vi "Event-Camera.vi"(5 "Menu ref.":refnum<k9>, 7 "Camera":T1, 8 "error in (no error)":errorcluster, 10 "Data ref. in":refnum<data-value>, 11 "UI ref. in":refnum<data-value>) -> (0 "error out":errorcluster, 2 "Data ref.":refnum<data-value>, 3 "UI ref.":refnum<data-value>)   [LabVIEW 2013, in "CameraVision.lvlib" / "CV-UI.lvclass"]
uses:
  CV-UI.lvclass
  Main/CV-Main.lvclass
  Camera-selector.ctl
  CV-UI.lvclass/CV-UI.ctl
  Main/Main-actions.ctl
  Read Camera.vi
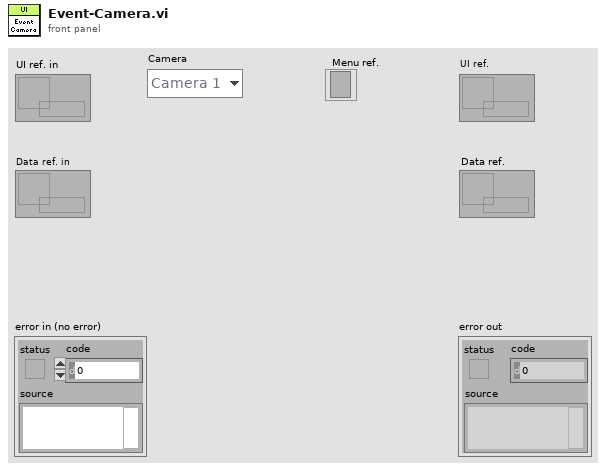
[diagram p1: front panel]
types:
  T1 = typedef "CameraVision.lvlib/CV-UI.lvclass/Camera-selector.ctl" = enum16{"Camera 1", "Camera 2"}
  T2 = typedef "CameraVision.lvlib/CV-Main.lvclass/Main-actions.ctl" = enum16{"Idle", "Initialize", "Load defaults", "Update settings", "Check settings", "Save settings", "Save settings with dialog", "Load settings", "Load data", "Activate", "Start", "Wait for start signal", "Acquire & process", "Iterate", "Stop", "Refresh display", "Refresh status", "View camera settings", "View grabber settings", "Exit"}
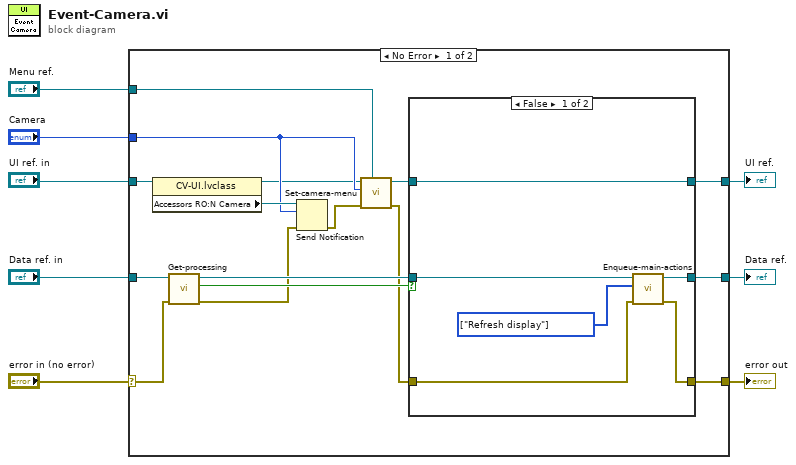
[diagram p0: block diagram]
diagram:
  n1 = case shown="No Error" "error in (no error)" {
    selector: "error in (no error)" -> [w18 w36]
    tunnel: [w17 w36] -> w7
    tunnel: [w20 w35] -> w5
    tunnel: "UI ref. in" -> [w23 w35]
    tunnel: "Data ref. in" -> [w24 w34]
    tunnel: "Camera" -> [w13 _]
    tunnel: [w19 w34] -> w2
    tunnel: "Menu ref." -> [w15 _]
    frame No Error {
      n2 = property class="CV-UI.lvclass"(reference=w23) -> (reference out=w9:refnum<data-value>, "Accessors RO:N Camera"=w14:refnum<notifier>)  [unwired: 1 in, 1 out]
      n3 = call "Get-processing.vi"("error in (no error)"=w18, "Data ref. in"=w24) -> ("error out"=w12:errorcluster, "Processing?"=w21:bool, "Data ref."=w22:refnum<data-value>)  [unwired: 7 in]
      n4 = Send Notification(notification=w13, notifier=w14, error in (no error)=w12) -> (error out=w11:errorcluster)  [unwired: 1 out]
      n5 = call "Set-camera-menu.vi"("Menu ref."=w15, "error in (no error)"=w11, "Camera in"=w13, "UI ref. in"=w9) -> ("error out"=w10:errorcluster, "UI ref."=w16:refnum<data-value>)  [unwired: 6 in]
      n6 = case shown="False" w21 {
        tunnel: w16 -> [w28 w32]
        tunnel: w22 -> [w26 w31]
        tunnel: [w28 w32] -> w20
        tunnel: [w25 w31] -> w19
        tunnel: w10 -> [w29 w33]
        tunnel: [w27 w33] -> w17
        frame False {
          w30 = T2[] [enum."Refresh display"] items=["Idle", "Initialize", "Load defaults", "Update settings", "Check settings", "Save settings", "Save settings with dialog", "Load settings", "Load data", "Activate", "Start", "Wait for start signal", "Acquire & process", "Iterate", "Stop", "Refresh display", "Refresh status", "View camera settings", "View grabber settings", "Exit"] ("State array")
          n7 = call "Enqueue-main-actions.vi"("error in (no error)"=w29, "State array"=w30, "Data ref. in"=w26) -> ("error out"=w27:errorcluster, "Data ref."=w25:refnum<data-value>)  [unwired: 6 in, 1 out]
        }
        frame True {
        }
      }
    }
    frame Error {
    }
  }
  "error out" <- w7
  "Data ref." <- w2
  "UI ref." <- w5
